vi "多参数测量数据存储.vi"(5 "数据类型":string(combo)="N", 6 "手动启动标记":bool, 7 "测量模式":T3(ring)=enum."水样测试", 8 "error in (no error)":errorcluster, 10 "table输入":string, 11 "data in":T2) -> (0 "error out":errorcluster)   [LabVIEW 2016, in "斯坦道多参数.lvlib"]
uses:
  <vilib>/Utility/error.llb/DialogType.ctl
  <vilib>/addons/database/Auxilliary.llb/DB Tools Column Info.ctl
  <vilib>/addons/database/Auxilliary.llb/DB Tools DataTypes.ctl
  <vilib>/addons/database/NI_Database_API.lvlib
panel:
  out "输出簇":T1
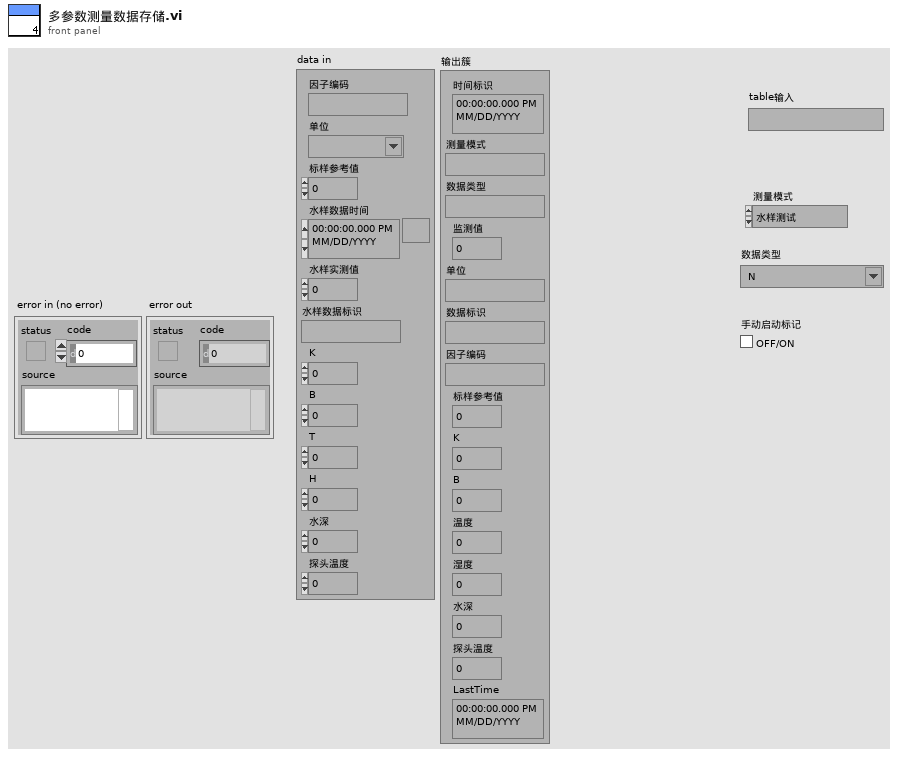
[diagram p1: front panel]
types:
  T1 = cluster{"时间标识":timestamp, "测量模式":string, "数据类型":string, "监测值":sgl, "单位":string, "数据标识":string, "因子编码":string, "标样参考值":sgl, "K":sgl, "B":sgl, "温度":sgl, "湿度":sgl, "水深":sgl, "探头温度":sgl, "LastTime":timestamp}
  T2 = cluster{"因子编码":string, "单位":string, "标样参考值":sgl, "水样数据时间":timestamp, "水样实测值":sgl, "水样数据标识":string, "K":sgl, "B":sgl, "T":sgl, "H":sgl, "水深":sgl, "探头温度":sgl}
  T3 = enum16{"待机", "水样测试", "标样核查", "零点核查", "跨度核查", "空白测试", "平行样测试", "加标回收", "空白校准", "标样校准", "初始化（清洗）"}
  T4 = typedef "NI_Database_API.lvlib/DB Tools Column Info.ctl" = cluster{"column name":string, "data type":T5, "size":i32, "allow null?":bool}
  T5 = typedef "NI_Database_API.lvlib/DB Tools DataTypes.ctl" = enum16{"String", "Long (I32)", "Single (SGL)", "Double (DBL)", "Date/Time", "Binary"}
  T6 = cluster{"时间标识":timestamp, "设备":string, "日志信息":string}
  T7 = typedef "DialogType.ctl" = u16
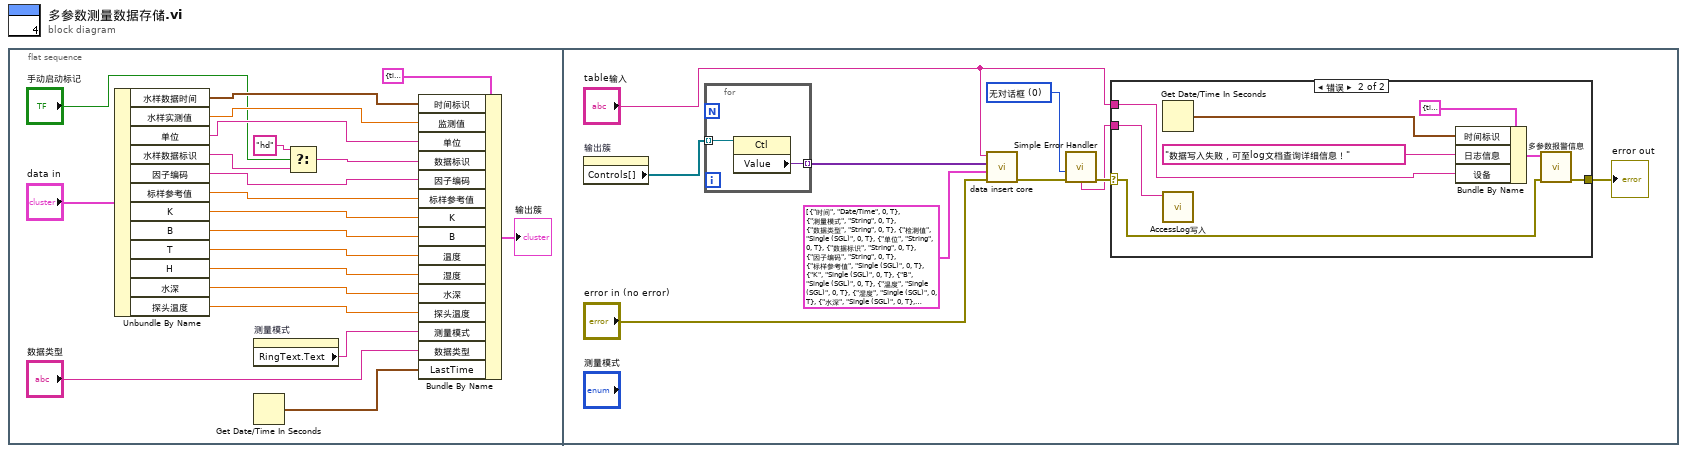
[diagram p0: block diagram]
diagram:
  n1 = flat-sequence {
    frame #0 {
      n2 = Unbundle By Name("data in") -> ("水样数据时间"=w21:timestamp, "水样实测值"=w20:sgl, "单位"=w14:string, "水样数据标识"=w1:string, "因子编码"=w13:string, "标样参考值"=w15:sgl, "K"=w16:sgl, "B"=w19:sgl, "T"=w18:sgl, "H"=w17:sgl, "水深"=w8:sgl, "探头温度"=w6:sgl)
      n3 = property on="测量模式" class="Enum (严格)"() -> ("RingText.Text"=w12:string)  [unwired: 2 in, 2 out]
      n4 = Get Date/Time In Seconds() -> (seconds since 1Jan1904=w5:timestamp)
      n5 = Select(t="hd", s="手动启动标记", f=w1) -> (s? t:f=w3:string)
      n6 = Bundle By Name(cluster=T1 {"时间标识"=timestamp(0 s since 1904-01-01), "测量模式"="", "数据类型"="", "监测值"=0.0, "单位"="", "数据标识"="", "因子编码"="", "标样参考值"=0.0, "K"=0.0, "B"=0.0, "温度"=0.0, "湿度"=0.0, "水深"=0.0, "探头温度"=0.0, "LastTime"=timestamp(0 s since 1904-01-01)} ("data输出"), "时间标识"=w21, "监测值"=w20, "单位"=w14, "数据标识"=w3, "因子编码"=w13, "标样参考值"=w15, "K"=w16, "B"=w19, "温度"=w18, "湿度"=w17, "水深"=w8, "探头温度"=w6, "测量模式"=w12, "数据类型"="数据类型", "LastTime"=w5) -> (→"输出簇":T1)
    }
    frame #1 {
      w22 = T7 0 items=["无对话框", "确定信息", "继续或停止信息", "确定信息＋警告", "继续/停止+警告"] ("type of dialog (OK msg:1)")
      n7 = property on="输出簇" class="Clust (严格)"() -> ("Controls[]"=w26:refnum<vi>[])  [unwired: 2 in, 2 out]
      n8 = for {
        tunnel: w26 -> [w33] mode=indexing
        tunnel: [w32] -> w27 mode=indexing
        n9 = property class="Ctl"(reference=w33) -> ("Value"=w32:variant)  [unwired: 1 in, 2 out]
      }
      n10 = call "data insert core.vi"("error in (no error)"="error in (no error)", "column information"=T4[] [{"column name"="时间", "data type"=enum."Date/Time", "size"=0, "allow null?"=TRUE}, {"column name"="测量模式", "data type"=enum."String", "size"=0, "allow null?"=TRUE}, {"column name"="数据类型", "data type"=enum."String", "size"=0, "allow null?"=TRUE}, {"column name"="检测值", "data type"=enum."Single (SGL)", "size"=0, "allow null?"=TRUE}, {"column name"="单位", "data type"=enum."String", "size"=0, "allow null?"=TRUE}, {"column name"="数据标识", "data type"=enum."String", "size"=0, "allow null?"=TRUE}, {"column name"="因子编码", "data type"=enum."String", "size"=0, "allow null?"=TRUE}, {"column name"="标样参考值", "data type"=enum."Single (SGL)", "size"=0, "allow null?"=TRUE}, {"column name"="K", "data type"=enum."Single (SGL)", "size"=0, "allow null?"=TRUE}, {"column name"="B", "data type"=enum."Single (SGL)", "size"=0, "allow null?"=TRUE}, {"column name"="温度", "data type"=enum."Single (SGL)", "size"=0, "allow null?"=TRUE}, {"column name"="湿度", "data type"=enum."Single (SGL)", "size"=0, "allow null?"=TRUE}, {"column name"="水深", "data type"=enum."Single (SGL)", "size"=0, "allow null?"=TRUE}, {"column name"="探头温度", "data type"=enum."Single (SGL)", "size"=0, "allow null?"=TRUE}, {"column name"="LastTime", "data type"=enum."Date/Time", "size"=0, "allow null?"=TRUE}], "data"=w27, "table"="table输入") -> ("error out"=w29:errorcluster)  [unwired: 7 in]
      n11 = call <vilib>:"Simple Error Handler.vi"("type of dialog (OK msg:1)"=w22, "error in (no error)"=w29) -> ("error out"=w24:errorcluster, "message"=w23:string)  [unwired: 3 in, 3 out]
      n12 = case shown="错误" w24 {
        selector: w24 -> [w34 w35]
        tunnel: w23 -> [_ w37]
        tunnel: [w34 w40] -> w25
        tunnel: "table输入" -> [_ w39]
        frame No Error {
        }
        frame Error {
          n13 = Get Date/Time In Seconds() -> (seconds since 1Jan1904=w38:timestamp)
          n14 = call "AccessLog写入.vi"("Log"=w37) -> ()  [unwired: 11 in]
          n15 = Bundle By Name(cluster=T6 {"时间标识"=timestamp(0 s since 1904-01-01), "设备"="", "日志信息"=""} ("data in"), "时间标识"=w38, "日志信息"="数据写入失败，可至log文档查询详细信息！", "设备"=w39) -> (w41:T6)
          n16 = call "多参数报警信息.vi"("error in (no error)"=w35, "data in"=w41) -> ("error out"=w40:errorcluster)  [unwired: 9 in]
        }
      }
      "error out" <- w25
    }
  }
